vi "GetWL_Back.vi"(2 "error in (no error)":errorcluster, 3 "Integration Time":i32, 4 "Type":T1, 5 "USB4000 Params In":T2) -> (0 "error out":errorcluster, 1 "USB4000 Params Out":T2)   [LabVIEW 2012]
uses:
  Controls/USB4000_Data.ctl
  Classes/Controls/SpectrometerOphirSelector.ctl
panel:
  out "EL spectrum":dbl[](array[numeric])
  out "Wavelength":dbl[](array[numeric]) format="%.2f"
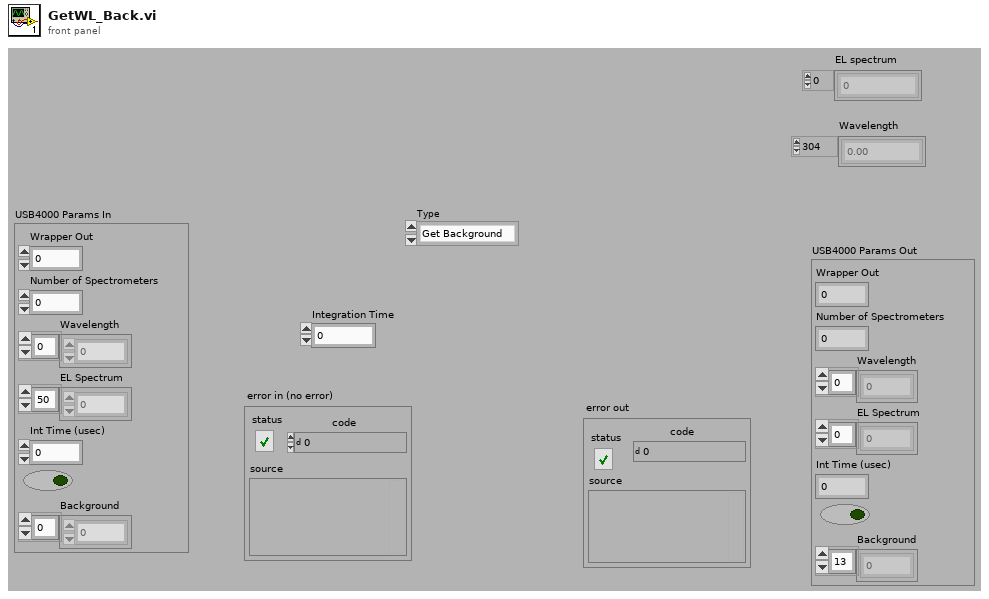
[diagram p1: front panel]
types:
  T1 = typedef "SpectrometerOphirSelector.ctl" = enum16{"Get Background", "Measure", "Measure50", "Raw"}
  T2 = typedef "USB4000_Data.ctl" = cluster{"Wrapper Out":u32, "Number of Spectrometers":i32, "Wavelength":dbl[], "EL Spectrum":dbl[], "Int Time (usec)":i32, bool, "Background":dbl[]}
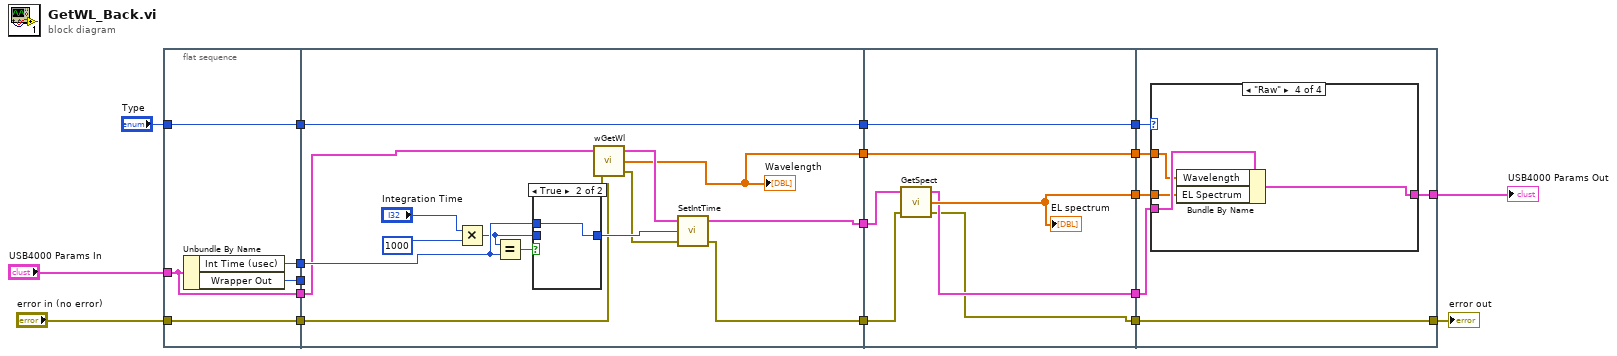
[diagram p0: block diagram]
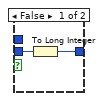
[diagram p2: hidden frame]
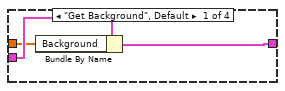
[diagram p3: hidden frame]
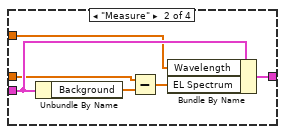
[diagram p4: hidden frame]
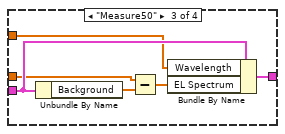
[diagram p5: hidden frame]
diagram:
  n1 = flat-sequence {
    tunnel: "error in (no error)" -> [w21]
    tunnel: [w23] -> w12
    tunnel: [w24] -> w11
    tunnel: [w21] -> w10
    tunnel: "USB4000 Params In" -> [w22]
    tunnel: [w22] -> w7
    tunnel: [w20] -> w3
    tunnel: "Type" -> [w20]
    tunnel: [w25] -> w19
    tunnel: [w27] -> w15
    tunnel: w12 -> [_]
    tunnel: w11 -> [w35]
    tunnel: w10 -> [w28]
    tunnel: w7 -> [w32]
    tunnel: [w33] -> w4
    tunnel: w3 -> [w33]
    tunnel: [w26] -> w1
    tunnel: w19 -> [w48]
    tunnel: [w48] -> w18
    tunnel: [w46] -> w17
    tunnel: [w42] -> w16
    tunnel: w15 -> [w43]
    tunnel: [w45] -> w8
    tunnel: [w47] -> w5
    tunnel: w4 -> [w47]
    tunnel: w1 -> [w44]
    tunnel: w18 -> [w54]
    tunnel: w17 -> [w53]
    tunnel: w16 -> [w52]
    tunnel: w8 -> [w50]
    tunnel: [w52] -> w6
    tunnel: [w51] -> w13
    tunnel: w5 -> [w49]
    frame #0 {
      n2 = Unbundle By Name(w22) -> ("Int Time (usec)"=w24:i32, "Wrapper Out"=w23:u32)
    }
    frame #1 {
      n3 = Multiply(x="Integration Time", y=1000) -> (x*y=w34:i32)
      n4 = Equal?(x=w34, y=w35) -> (x = y?=w36:bool)
      n5 = case shown="True" w36 {
        tunnel: [w39 w41] -> w31
        tunnel: w35 -> [_ w41]
        tunnel: w34 -> [w40 _]
        frame False {
          n6 = To Long Integer(number=w40) -> (32bit integer=w39:i32)
        }
        frame True {
        }
      }
      n7 = call "wGetWl.vi"("error in (no error)"=w28, "SpectRef In"=w32) -> ("error out"=w29:errorcluster, "WL Values"=w25:dbl[], "SpectRef Out"=w30:T2)  [unwired: 1 in]
      "Wavelength" <- w25
      n8 = call "SetIntTime.vi"("error in"=w29, "Integration Time"=w31, "SpectRef In"=w30) -> ("error out"=w27:errorcluster, "SpectRef Out"=w26:T2)  [unwired: 1 in]
    }
    frame #2 {
      n9 = call "GetSpect.vi"("error in (no error)"=w43, "SpectRef In"=w44) -> ("error out"=w42:errorcluster, "Spectrum Values"=w46:dbl[], "SpectRef Out"=w45:T2)  [unwired: 1 in]
      "EL spectrum" <- w46
    }
    frame #3 {
      n10 = case shown="\"Raw\"" w49 {
        tunnel: w50 -> [w57 w63 w69 w72]
        tunnel: w54 -> [_ w58 w64 w71]
        tunnel: w53 -> [w56 w61 w67 w70]
        tunnel: [w55 w59 w65 w73] -> w51
        frame "Get Background", Default {
          n11 = Bundle By Name(cluster=w57, "Background"=w56) -> (w55:T2)
        }
        frame "Measure" {
          n12 = Unbundle By Name(w63) -> ("Background"=w62:dbl[])
          n13 = Subtract(x=w61, y=w62) -> (x-y=w60:dbl[])
          n14 = Bundle By Name(cluster=w63, "Wavelength"=w58, "EL Spectrum"=w60) -> (w59:T2)
        }
        frame "Measure50" {
          n15 = Unbundle By Name(w69) -> ("Background"=w68:dbl[])
          n16 = Subtract(x=w67, y=w68) -> (x-y=w66:dbl[])
          n17 = Bundle By Name(cluster=w69, "Wavelength"=w64, "EL Spectrum"=w66) -> (w65:T2)
        }
        frame "Raw" {
          n18 = Bundle By Name(cluster=w72, "Wavelength"=w71, "EL Spectrum"=w70) -> (w73:T2)
        }
      }
    }
  }
  "USB4000 Params Out" <- w13
  "error out" <- w6
